vi "0721_Controle_FMS.vi"() -> ()   [LabVIEW 2017]
uses:
  <vilib>/myRIO/Instrument Drivers/Onboard IO/PWM/typedefs/PWM Reference.ctl
  <vilib>/myRIO/Common/Instrument Driver Framework/Utilities/typedefs/myRIO Generic Hardware Reference.ctl
  <vilib>/myRIO/Common/Instrument Driver Framework/Utilities/typedefs/Hardware Version Enum.ctl
  <vilib>/myRIO/Common/Instrument Driver Framework/Utilities/typedefs/myRIO v1.0 Reference.ctl
  <vilib>/myRIO/Common/Instrument Driver Framework/Utilities/typedefs/Generic FPGA Reference.ctl
  <vilib>/myRIO/Common/Instrument Driver Framework/myRIO v1.0/PWM/typedefs/PWM Channels Enum.ctl
  <vilib>/myRIO/Instrument Drivers/Onboard IO/PWM/typedefs/PWM Configuration.ctl
  <vilib>/userdefined/High Color/nirio_resource_hc.ctl
  <vilib>/myRIO/Common/Instrument Driver Framework/myRIO v1.0/PWM/vis/myRIO v1.1 Open PWM.vi
  <vilib>/myRIO/Common/Instrument Driver Framework/Utilities/vis/Validate Channels.vi
  <vilib>/myRIO/Common/Instrument Driver Framework/myRIO v1.0/PWM/vis/myRIO v1.0 Reserve PWM.vi
  <vilib>/myRIO/Instrument Drivers/Onboard IO/PWM/vis/Set Duty Cycle and Frequency.vi
  <vilib>/myRIO/Common/Instrument Driver Framework/myRIO v1.0/PWM/vis/myRIO v1.0 Close PWM.vi
  <vilib>/myRIO/Common/Instrument Driver Framework/myRIO v1.0/PWM/vis/myRIO v1.0 Build MUX Configuration PWM.vi
  <vilib>/myRIO/Common/Instrument Driver Framework/myRIO v1.0/Resource Manager/vis/myRIO v1.0 Reserve Channel List.vi
  <vilib>/myRIO/Common/Instrument Driver Framework/myRIO v1.0/PWM/vis/myRIO v1.0 Unreserve PWM.vi
  <vilib>/myRIO/Common/Instrument Driver Framework/myRIO v1.0/Resource Manager/vis/myRIO v1.0 Create Configuration List.vi
  <vilib>/myRIO/Common/Instrument Driver Framework/myRIO v1.0/Resource Manager/vis/myRIO v1.0 Reserve Channel.vi
  <vilib>/myRIO/Common/Instrument Driver Framework/myRIO v1.0/Resource Manager/vis/myRIO v1.0 Unreserve Channel.vi
  <vilib>/myRIO/Common/Instrument Driver Framework/myRIO v1.0/Resource Manager/vis/myRIO v1.0 Unreserve Channel List.vi
  <vilib>/myRIO/Common/Instrument Driver Framework/myRIO v1.0/Resource Manager/vis/myRIO v1.0 Build Mutex Name.vi
  <vilib>/Utility/VariantDataType/GetNumericInfo.vi
  <vilib>/Utility/error.llb/Error Cluster From Error Code.vi
  <vilib>/myRIO/Common/Instrument Driver Framework/myRIO v1.0/myRIO v1.1 Open.vi
  <vilib>/myRIO/Common/Instrument Driver Framework/Utilities/vis/IO Manager.vi
  <vilib>/myRIO/Common/Instrument Driver Framework/Utilities/vis/Configuration Manager.vi
  <vilib>/myRIO/Common/Instrument Driver Framework/myRIO v1.0/Resource Manager/vis/myRIO v1.0 Configure IO.vi
  <vilib>/myRIO/Common/Instrument Driver Framework/myRIO v1.0/myRIO v1.0 Close.vi
  <vilib>/myRIO/Common/Instrument Driver Framework/myRIO v1.0/PWM/vis/myRIO v1.0 Write PWM.vi
  <vilib>/myRIO/Common/Instrument Driver Framework/myRIO v1.0/PWM/vis/myRIO v1.0 Shutdown PWM.vi
  <vilib>/myRIO/Instrument Drivers/Onboard IO/PWM/vis/myRIO PWM Open.xnode
  <vilib>/myRIO/Instrument Drivers/Onboard IO/PWM/PWM.lvlib
panel:
  in  "Posições_peça":u16(ring) items=["Local A", "Local B", "Local C"]
  in  "delay between positions (ms)":u32=5
  out "Manipulating":bool
  out "Ready_to_manipulate":bool
  out "Is_position_desired":bool
  out "Is_robot_home":bool
  out "Local_stop":bool
  out "ms":u32
  in  "Stop conveyor":bool=TRUE
  in  "Conveyor speed (mm/s)":dbl(slide)=200.0 step=1.0 scale=0.0..350.0
  in  "Actuator":bool
  in  "Positions_control":u16(ring) items=["Livre", "Posição 1", "Posição 2", "Posição 3", "Posição 4", "Posição 5", "Posição 6", "Posição 7", "Fim"]
  in  "Stop":bool
  out "Position":dbl[](array[knob]) scale=0.0..200.0
  in  "Desired position":dbl[](array[slide])=[150.0, 0.0, 100.0, 100.0, 100.0, 100.0] min=0.0 max=180.0 step=1.0 scale=0.0..180.0
  in  "Home":bool
  out "error out":errorcluster
  in  "error in (no error)":errorcluster
  in  "ms to wait (braço)":u32=5
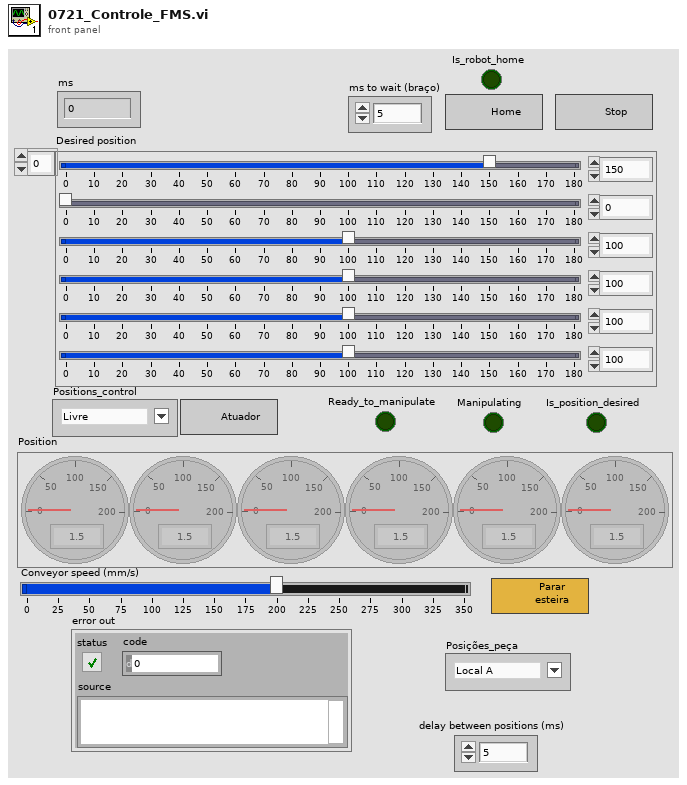
[diagram p1: front panel]
types:
  T1 = typedef "nirio_resource_hc.ctl" = tag
  T2 = typedef "Hardware Version Enum.ctl" = enum16{"Unknown", "myRIO-1900", "myRIO-1950", "roboRIO", "NI ELVIS RIO CM"}
  T3 = typedef "PWM.lvlib/PWM Reference.ctl" = cluster{"myRIO Reference":T4, "PWM Channels Enum":T7, "PWM Configuration":T8}
  T4 = typedef "myRIO Generic Hardware Reference.ctl" = cluster{"myRIO Model":T2, "myRIO Hardware Reference":T5}
  T5 = typedef "myRIO v1.0 Reference.ctl" = cluster{"Generic FPGA Reference":T6, "Allow multiple opens":bool}
  T6 = typedef "Generic FPGA Reference.ctl" = refnum<k20>
  T7 = typedef "PWM Channels Enum.ctl" = enum16{"Not Connected", "C/PWM0", "C/PWM1", "A/PWM0", "A/PWM1", "A/PWM2", "B/PWM0", "B/PWM1", "B/PWM2", "PWM/PWM0", "PWM/PWM1", "PWM/PWM2", "PWM/PWM3", "PWM/PWM4", "PWM/PWM5", "PWM/PWM6", "PWM/PWM7", "PWM/PWM8", "PWM/PWM9"}
  T8 = typedef "PWM.lvlib/PWM Configuration.ctl" = cluster{"Frequency":dbl, "Duty Cycle":dbl}
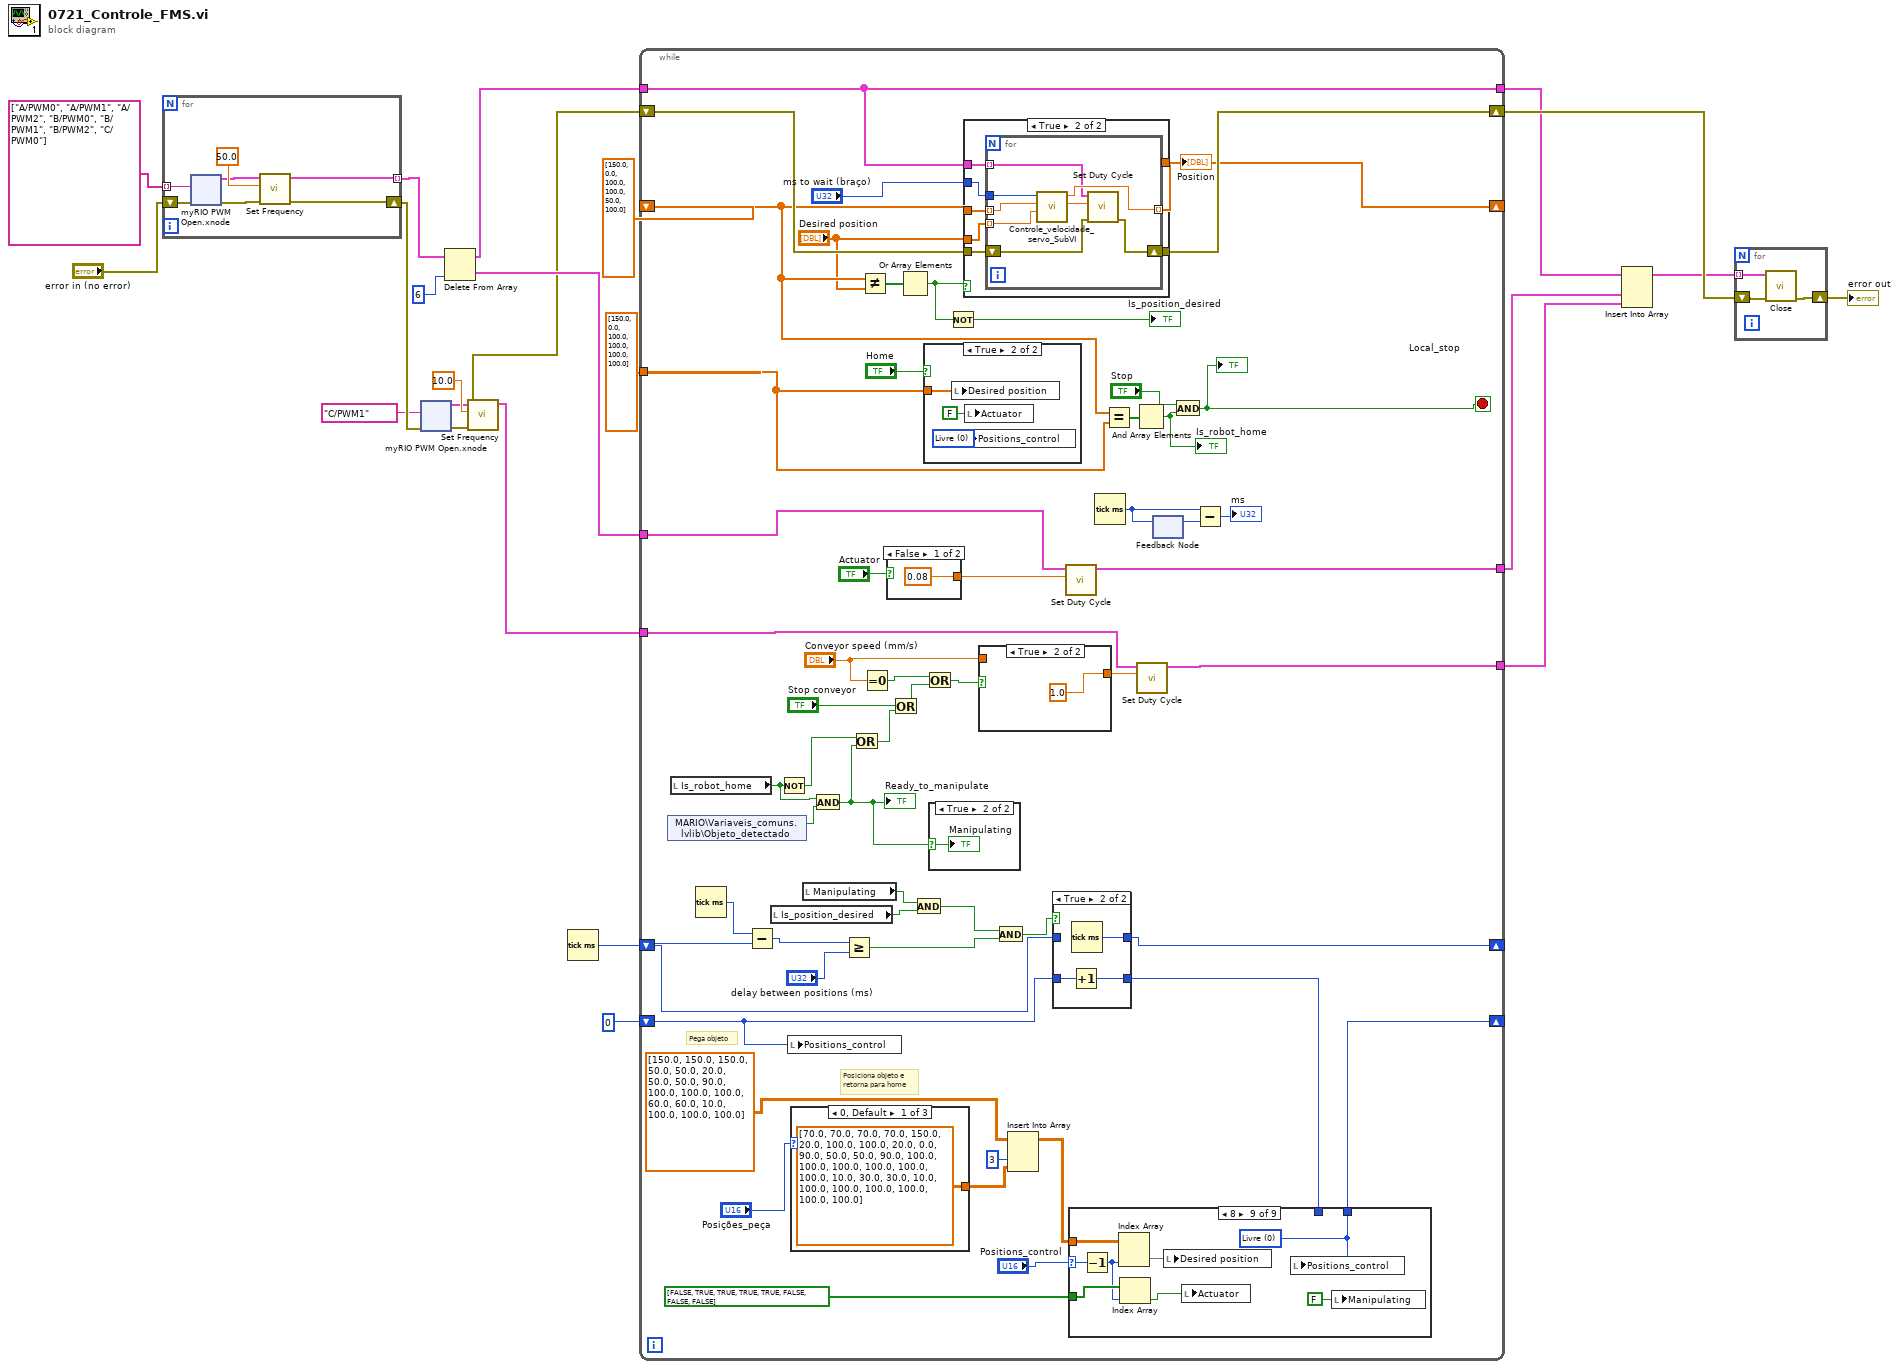
[diagram p0: block diagram]
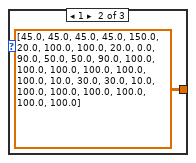
[diagram p2: hidden frame]
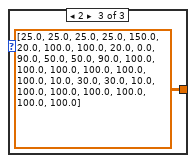
[diagram p3: hidden frame]
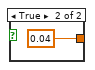
[diagram p7: hidden frame]
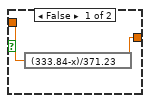
[diagram p9: hidden frame]
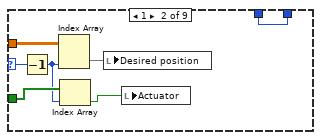
[diagram p11: hidden frame]
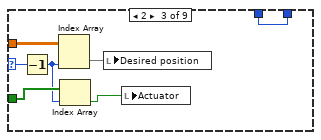
[diagram p12: hidden frame]
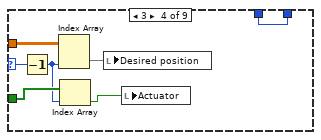
[diagram p13: hidden frame]
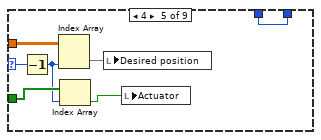
[diagram p14: hidden frame]
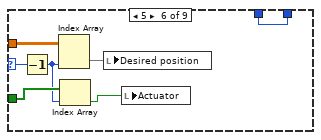
[diagram p15: hidden frame]
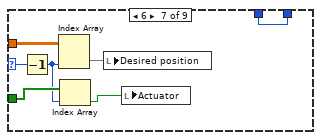
[diagram p16: hidden frame]
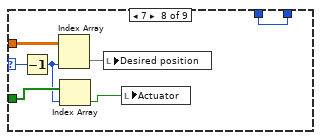
[diagram p17: hidden frame]
diagram:
  n1 = for {
    shift-right: [w24] -> w13
    shift-left: "error in (no error)" -> [w29]
    tunnel: tag[] ["A/PWM0", "A/PWM1", "A/PWM2", "B/PWM0", "B/PWM1", "B/PWM2", "C/PWM0"] -> [w30] mode=indexing
    tunnel: [w25] -> w10 mode=indexing
    n2 = xnode "myRIO PWM Open.xnode"("error in (no error)"=w29, "Channel Name"=w30) -> ("error out"=w27:errorcluster, "PWM Ref Out"=w26:T3)  [unwired: 1 in]
    n3 = call <vilib>:"Set Frequency.vi"("error in (no error)"=w27, "Frequency [Hz]"=50.0, "PWM Ref In"=w26) -> ("error out"=w24:errorcluster, "PWM Ref Out"=w25:T3)  [unwired: 6 in]
  }
  n4 = xnode "myRIO PWM Open.xnode"("error in (no error)"=w13, "Channel Name"=tag "C/PWM1") -> ("error out"=w14:errorcluster, "PWM Ref Out"=w15:T3)  [unwired: 1 in]
  n5 = Delete From Array(array=w10, index=6) -> (deleted portion=w7:T3, array with subset deleted=w8:T3[])  [unwired: 1 in]
  n6 = call <vilib>:"Set Frequency.vi"("error in (no error)"=w14, "Frequency [Hz]"=10.0, "PWM Ref In"=w15) -> ("error out"=w6:errorcluster, "PWM Ref Out"=w5:T3)  [unwired: 6 in]
  n7 = Tick Count (ms)() -> (millisecond timer value=w2:u32)
  n8 = while {
    shift-right: [w100] -> w23
    shift-left: w6 -> [w101]
    shift-right: [w99] -> _
    shift-left: dbl[] [150.0, 0.0, 100.0, 100.0, 50.0, 100.0] -> [w81]
    tunnel: w8 -> [w98]
    tunnel: [w98] -> w20
    tunnel: dbl[] [150.0, 0.0, 100.0, 100.0, 100.0, 100.0] -> [w94]
    tunnel: w7 -> [w92]
    tunnel: [w90] -> w19
    tunnel: w5 -> [w88]
    tunnel: [w86] -> w17
    shift-right: [w59] -> _
    shift-left: w2 -> [w60]
    shift-right: [w56] -> _
    shift-left: 0 -> [w58]
    stop <- w78 stop-if-true
    # "Posiciona objeto e \nretorna para home"
    # "Pega objeto"
    n9 = shared-variable "MARIO\\Variaveis_comuns.lvlib\\Objeto_detectado"() -> (w73:bool)  [unwired: 1 in, 1 out]
    n10 = local read "Is_robot_home"() -> (w72:bool)
    n11 = Tick Count (ms)() -> (millisecond timer value=w64:u32)
    n12 = Subtract(x=w64, y=w60) -> (x-y=w63:u32)
    n13 = local read "Is_position_desired"() -> (w54:bool)
    n14 = Not(x=w72) -> (.not. x?=w71:bool)
    n15 = local write "Positions_control"(w58) -> ()
    n16 = case shown="0, Default" "Posições_peça" {
      tunnel: [dbl[][] [[70.0, 70.0, 70.0, 70.0, 150.0], [20.0, 100.0, 100.0, 20.0, 0.0], [90.0, 50.0, 50.0, 90.0, 100.0], [100.0, 100.0, 100.0, 100.0, 100.0], [10.0, 30.0, 30.0, 10.0, 100.0], [100.0, 100.0, 100.0, 100.0, 100.0]] ("Positions") dbl[][] [[45.0, 45.0, 45.0, 45.0, 150.0], [20.0, 100.0, 100.0, 20.0, 0.0], [90.0, 50.0, 50.0, 90.0, 100.0], [100.0, 100.0, 100.0, 100.0, 100.0], [10.0, 30.0, 30.0, 10.0, 100.0], [100.0, 100.0, 100.0, 100.0, 100.0]] ("Positions") dbl[][] [[25.0, 25.0, 25.0, 25.0, 150.0], [20.0, 100.0, 100.0, 20.0, 0.0], [90.0, 50.0, 50.0, 90.0, 100.0], [100.0, 100.0, 100.0, 100.0, 100.0], [10.0, 30.0, 30.0, 10.0, 100.0], [100.0, 100.0, 100.0, 100.0, 100.0]] ("Positions")] -> w49
      frame 0, Default {
      }
      frame 1 {
      }
      frame 2 {
      }
    }
    n17 = local read "Manipulating"() -> (w55:bool)
    n18 = And(x=w72, y=w73) -> (x .and. y?=w66:bool)
    "Ready_to_manipulate" <- w66
    n19 = Greater Or Equal?(x=w63, y="delay between positions (ms)") -> (x >= y?=w62:bool)
    n20 = Or(x=w71, y=w66) -> (x .or. y?=w70:bool)
    n21 = Not Equal?(x=w81, y="Desired position") -> (x != y?=w79:bool[])
    n22 = Equal To 0?(x="Conveyor speed (mm/s)") -> (x = 0?=w77:bool)
    n23 = case shown="False" "Actuator" {
      tunnel: [0.08 ("Duty Cycle Abert") 0.04 ("Duty Cycle Abert")] -> w91
      frame False {
      }
      frame True {
      }
    }
    n24 = Or(x="Stop conveyor", y=w70) -> (x .or. y?=w75:bool)
    n25 = Or Array Elements(Boolean array=w79) -> (logical OR=w69:bool)
    n26 = And(x=w55, y=w54) -> (x .and. y?=w53:bool)
    n27 = case shown="True" "Home" {
      tunnel: w94 -> [_ w133]
      frame False {
      }
      frame True {
        w131 = u16 0 items=["Livre", "Posição 1", "Posição 2", "Posição 3", "Posição 4", "Posição 5"] ("Menu Ring")
        n28 = local write "Desired position"(w133) -> ()
        n29 = local write "Positions_control"(w131) -> ()
        n30 = local write "Actuator"(FALSE ("Atuador")) -> ()
      }
    }
    n31 = Or(x=w77, y=w75) -> (x .or. y?=w85:bool)
    n32 = case shown="True" w66 {
      selector: w66 -> [_ w111]
      frame False {
      }
      frame True {
        "Manipulating" <- w111
      }
    }
    n33 = Not(x=w69) -> (.not. x?=→"Is_position_desired":bool)
    n34 = case shown="True" w69 {
      tunnel: "ms to wait (braço)" -> [_ w120]
      tunnel: "Desired position" -> [_ w119]
      tunnel: w101 -> [w113 w118]
      tunnel: [w113 w117] -> w100
      tunnel: [w112 w116] -> w99
      tunnel: w98 -> [_ w115]
      tunnel: w81 -> [w112 w114]
      frame False {
      }
      frame True {
        n35 = for {
          tunnel: w120 -> [w128]
          tunnel: w115 -> [w123] mode=indexing
          tunnel: w119 -> [w121] mode=indexing
          tunnel: w114 -> [w122] mode=indexing
          shift-right: [w124] -> w117
          shift-left: w118 -> [w125]
          tunnel: [w127] -> w116 mode=indexing
          n36 = call "Controle_velocidade_servo_SubVI.vi"("Posição Desejada"=w121, "Posição"=w122, "milliseconds to wait"=w128) -> ("Duty Cycle"=w126:dbl, "Posição"=w127:dbl)  [unwired: 7 in]
          n37 = call <vilib>:"Set Duty Cycle.vi"("error in (no error)"=w125, "Duty Cycle"=w126, "PWM Ref In"=w123) -> ("error out"=w124:errorcluster)  [unwired: 6 in, 1 out]
        }
      }
    }
    "Position" <- w99
    n38 = case shown="True" w85 {
      tunnel: [w134 1.0] -> w87
      tunnel: "Conveyor speed (mm/s)" -> [w135 _]
      frame False {
        n39 = expression code="(333.84-x)/371.23"(w135) -> (w134:dbl)
      }
      frame True {
      }
    }
    n40 = And(x=w53, y=w62) -> (x .and. y?=w61:bool)
    n41 = Insert Into Array(array=dbl[][] [[150.0, 150.0, 150.0], [50.0, 50.0, 20.0], [50.0, 50.0, 90.0], [100.0, 100.0, 100.0], [60.0, 60.0, 10.0], [100.0, 100.0, 100.0]] ("Positions"), index (col)=3 ("disabled index (col)"), new element=w49) -> (w48:dbl[][])  [unwired: 1 in]
    n42 = case shown="True" w61 {
      tunnel: w60 -> [w107 _]
      tunnel: [w107 w110] -> w59
      tunnel: w58 -> [w106 w109]
      tunnel: [w106 w108] -> w57
      frame False {
      }
      frame True {
        n43 = Increment(x=w109) -> (x+1=w108:i32)
        n44 = Tick Count (ms)() -> (millisecond timer value=w110:u32)
      }
    }
    n45 = call <vilib>:"Set Duty Cycle.vi"("Duty Cycle"=w91, "PWM Ref In"=w92) -> ("PWM Ref Out"=w90:T3)  [unwired: 7 in, 1 out]
    n46 = case shown="8" "Positions_control" {
      selector: "Positions_control" -> [_ w142 w149 w156 w163 w170 w177 w184 w192]
      tunnel: w48 -> [_ w144 w151 w158 w165 w172 w179 w186 w194]
      tunnel: bool[] [FALSE, TRUE, TRUE, TRUE, TRUE, FALSE, FALSE, FALSE] ("Actuator_positions") -> [_ w141 w148 w155 w162 w169 w176 w183 w191]
      tunnel: w57 -> [w137 w138 w145 w152 w159 w166 w173 w180 _]
      tunnel: [w137 w138 w145 w152 w159 w166 w173 w180 w187] -> w56
      frame 0, Default {
      }
      frame 1 {
        n47 = Decrement(x=w142) -> (x-1=w140:u16)
        n48 = Index Array(array=w144, index (col)=w140) -> (element=w143:dbl[])  [unwired: 1 in]
        n49 = Index Array(array=w141, index=w140) -> (element=w139:bool)
        n50 = local write "Desired position"(w143) -> ()
        n51 = local write "Actuator"(w139) -> ()
      }
      frame 2 {
        n52 = Decrement(x=w149) -> (x-1=w147:u16)
        n53 = Index Array(array=w151, index (col)=w147) -> (element=w150:dbl[])  [unwired: 1 in]
        n54 = Index Array(array=w148, index=w147) -> (element=w146:bool)
        n55 = local write "Desired position"(w150) -> ()
        n56 = local write "Actuator"(w146) -> ()
      }
      frame 3 {
        n57 = Decrement(x=w156) -> (x-1=w154:u16)
        n58 = Index Array(array=w158, index (col)=w154) -> (element=w157:dbl[])  [unwired: 1 in]
        n59 = Index Array(array=w155, index=w154) -> (element=w153:bool)
        n60 = local write "Desired position"(w157) -> ()
        n61 = local write "Actuator"(w153) -> ()
      }
      frame 4 {
        n62 = Decrement(x=w163) -> (x-1=w161:u16)
        n63 = Index Array(array=w165, index (col)=w161) -> (element=w164:dbl[])  [unwired: 1 in]
        n64 = Index Array(array=w162, index=w161) -> (element=w160:bool)
        n65 = local write "Desired position"(w164) -> ()
        n66 = local write "Actuator"(w160) -> ()
      }
      frame 5 {
        n67 = Decrement(x=w170) -> (x-1=w168:u16)
        n68 = Index Array(array=w172, index (col)=w168) -> (element=w171:dbl[])  [unwired: 1 in]
        n69 = Index Array(array=w169, index=w168) -> (element=w167:bool)
        n70 = local write "Desired position"(w171) -> ()
        n71 = local write "Actuator"(w167) -> ()
      }
      frame 6 {
        n72 = Decrement(x=w177) -> (x-1=w175:u16)
        n73 = Index Array(array=w179, index (col)=w175) -> (element=w178:dbl[])  [unwired: 1 in]
        n74 = Index Array(array=w176, index=w175) -> (element=w174:bool)
        n75 = local write "Desired position"(w178) -> ()
        n76 = local write "Actuator"(w174) -> ()
      }
      frame 7 {
        n77 = Decrement(x=w184) -> (x-1=w182:u16)
        n78 = Index Array(array=w186, index (col)=w182) -> (element=w185:dbl[])  [unwired: 1 in]
        n79 = Index Array(array=w183, index=w182) -> (element=w181:bool)
        n80 = local write "Desired position"(w185) -> ()
        n81 = local write "Actuator"(w181) -> ()
      }
      frame 8 {
        w187 = u16 0 items=["Livre", "Posição 1", "Posição 2", "Posição 3", "Posição 4", "Posição 5", "Posição 6", "Posição 7", "Fim"] ("Positions_control")
        n82 = Decrement(x=w192) -> (x-1=w190:u16)
        n83 = Index Array(array=w194, index (col)=w190) -> (element=w193:dbl[])  [unwired: 1 in]
        n84 = Index Array(array=w191, index=w190) -> (element=w189:bool)
        n85 = local write "Desired position"(w193) -> ()
        n86 = local write "Actuator"(w189) -> ()
        n87 = local write "Positions_control"(w187) -> ()
        n88 = local write "Manipulating"(FALSE ("Manipulating")) -> ()
      }
    }
    n89 = Tick Count (ms)() -> (millisecond timer value=w83:u32)
    n90 = Equal?(x=w81, y=w94) -> (x = y?=w95:bool[])
    n91 = And Array Elements(Boolean array=w95) -> (logical AND=w74:bool)
    "Is_robot_home" <- w74
    n92 = call <vilib>:"Set Duty Cycle.vi"("Duty Cycle"=w87, "PWM Ref In"=w88) -> ("PWM Ref Out"=w86:T3)  [unwired: 7 in, 1 out]
    n93 = feedback-in #1(w83) -> ()
    n94 = feedback #1() -> (w82:u32)  [unwired: 1 in]
    n95 = And(x="Stop", y=w74) -> (x .and. y?=w78:bool)
    "Local_stop" <- w78
    n96 = Subtract(x=w83, y=w82) -> (x-y=→"ms":u32)
  }
  n97 = Insert Into Array(array=w20, new element #1=w19, new element #2=w17) -> (w18:T3[])  [unwired: 1 in]
  n98 = for {
    tunnel: w18 -> [w197] mode=indexing
    shift-right: [w195] -> w22
    shift-left: w23 -> [w196]
    n99 = call <vilib>:"Close.vi"("error in (no error)"=w196, "PWM Ref In"=w197) -> ("error out"=w195:errorcluster)  [unwired: 9 in]
  }
  "error out" <- w22
